vi "PiezoDAQStart.vi"(3 "Waveform":waveform(dbl)={"t0"=timestamp(0 s since 1904-01-01), "dt"=0.0, "Y"=[]}, 10 "error in (no error)":errorcluster) -> (6 "error out":errorcluster)   [LabVIEW 2009]
uses:
  PiezoGlobal.vi
  <vilib>/DAQmx/configure/trigger.llb/DAQmx Start Trigger (Digital Edge).vi
  <vilib>/DAQmx/create/channels.llb/DAQmx Create Channel (CO-Pulse Generation-Time).vi
  <vilib>/DAQmx/configure/timing.llb/DAQmx Timing (Implicit).vi
  <vilib>/DAQmx/write.llb/DAQmx Write (Analog Wfm 1Chan NSamp).vi
  <vilib>/DAQmx/configure/timing.llb/DAQmx Timing (Sample Clock).vi
  <vilib>/DAQmx/create/channels.llb/DAQmx Create Channel (AO-Voltage-Basic).vi
  <vilib>/Waveform/WDTOps.llb/WDT Number of Waveform Samples DBL.vi
  Program Files/National Instruments/LabVIEW 2009/resource/objmgr/daqmx.rc
panel:
  out "True Base Time":dbl format="%.6g"
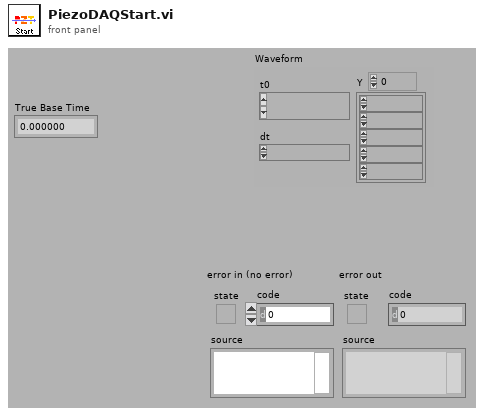
[diagram p1: front panel]
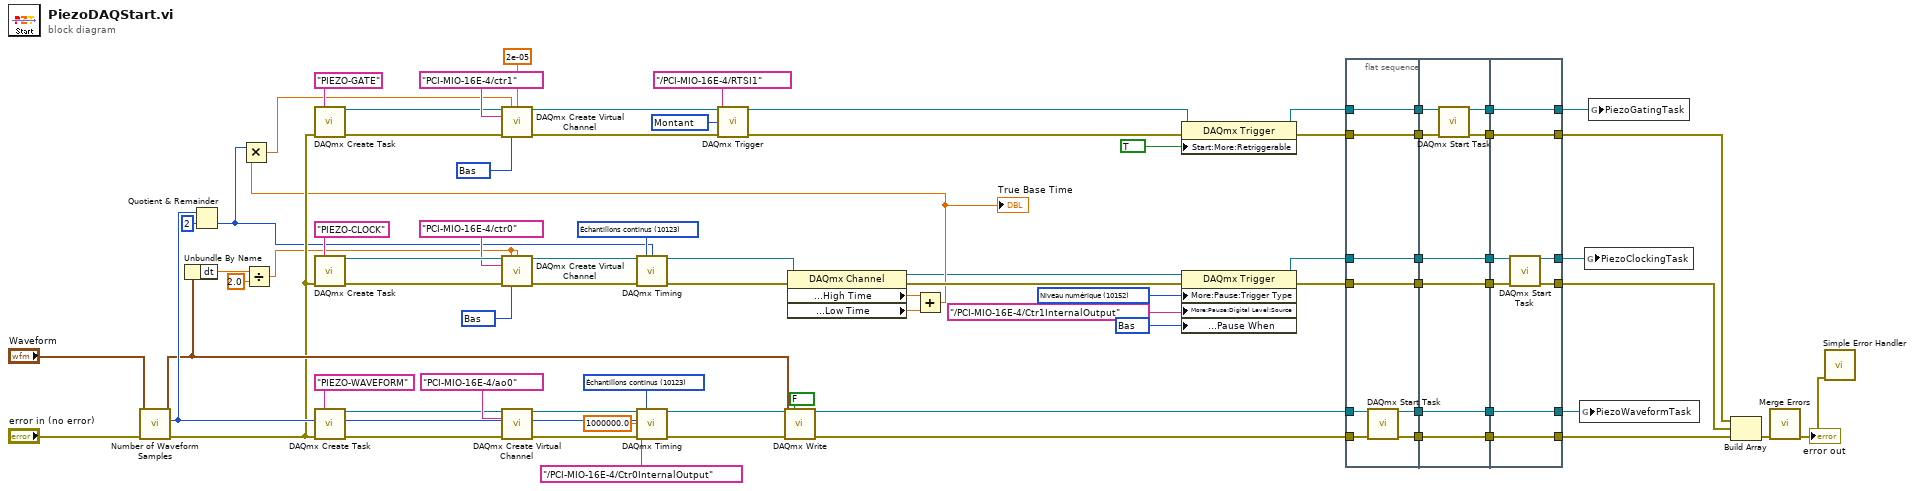
[diagram p0: block diagram]
diagram:
  w32 = 10214 items=["Haut"=10192, "Bas"=10214] ("idle state")
  w33 = 10214 items=["Haut"=10192, "Bas"=10214] ("idle state")
  w38 = 10214 items=["Haut"=10192, "Bas"=10214] ("Pause.NivNum.Lors")
  w39 = 10152 items=["Niveau analogique"=10101, "Fenêtre analogique"=10103, "Niveau numérique"=10152, "Pattern numérique"=10398, "Aucun"=10230] ("Pause.TypeDécl")
  w46 = 10280 items=["Montant"=10280, "Descendant"=10171] ("edge")
  w68 = 10123 items=["Échantillons finis"=10178, "Échantillons continus"=10123, "Point par point avec cadencement matériel"=12522] ("sample mode")
  w77 = 10123 items=["Échantillons finis"=10178, "Échantillons continus"=10123, "Point par point avec cadencement matériel"=12522] ("sample mode")
  n1 = call-poly <vilib>:"Number of Waveform Samples.vi"("error in (no error)"="error in (no error)", "waveform in"="Waveform") -> ("error out"=w36:errorcluster, "number of samples"=w67:i32, "waveform out"=w37:waveform(dbl))  [unwired: 7 in]
  n2 = Unbundle By Name(w37) -> ("dt"=w10:dbl)
  n3 = Quotient & Remainder(x=w67, y=2) -> (floor(x/y)=w19:i32)  [unwired: 1 out]
  n4 = Divide(x=w10, y=2.0) -> (x/y=w8:dbl)
  n5 = call <vilib>:"DAQmx Create Task.vi"("new task name"="PIEZO-GATE", "error in"=w36) -> ("task out"=w50:refnum<k21>, "error out"=w51:errorcluster)  [unwired: 12 in]
  n6 = call <vilib>:"DAQmx Create Task.vi"("new task name"="PIEZO-CLOCK", "error in"=w36) -> ("task out"=w79:refnum<k21>, "error out"=w78:errorcluster)  [unwired: 12 in]
  n7 = call <vilib>:"DAQmx Create Task.vi"("new task name"="PIEZO-WAVEFORM", "error in"=w36) -> ("task out"=w3:refnum<k21>, "error out"=w73:errorcluster)  [unwired: 12 in]
  n8 = call-poly <vilib>:"DAQmx Create Virtual Channel.vi"("task in"=w79, "high time"=w8, "low time"=w8, "counter"=tag "PCI-MIO-16E-4/ctr0", "error in"=w78, "idle state"=w32) -> ("task out"=w57:refnum<k21>, "error out"=w75:errorcluster)  [unwired: 8 in]
  n9 = call-poly <vilib>:"DAQmx Create Virtual Channel.vi"("task in"=w3, "physical channels"=tag "PCI-MIO-16E-4/ao0", "error in"=w73) -> ("task out"=w69:refnum<k21>, "error out"=w70:errorcluster)  [unwired: 11 in]
  n10 = call-poly <vilib>:"DAQmx Timing.vi"("task/channels in"=w57, "sample mode"=w77, "samples per channel"=w19, "error in"=w75) -> ("task out"=w13:refnum<k21>, "error out"=w15:errorcluster)  [unwired: 10 in]
  n11 = call-poly <vilib>:"DAQmx Timing.vi"("task/channels in"=w69, "sample mode"=w68, "samples per channel"=w67, "rate"=1000000.0, "source"=tag "/PCI-MIO-16E-4/Ctr0InternalOutput", "error in"=w70) -> ("task out"=w65:refnum<k21>, "error out"=w66:errorcluster)  [unwired: 8 in]
  n12 = call-poly <vilib>:"DAQmx Write.vi"("task/channels in"=w65, "auto start"=FALSE, "data"=w37, "error in"=w66) -> ("task out"=w1:refnum<k21>, "error out"=w2:errorcluster)  [unwired: 9 in, 1 out]
  n13 = property class="DAQmx Channel"(reference=w13, error in=w15) -> (reference out=w5:refnum<k21>, error out=w14:errorcluster, "Counter Output:Pulse:Time:High Time"=w12:dbl, "Counter Output:Pulse:Time:Low Time"=w11:dbl)
  n14 = Add(x=w12, y=w11) -> (x+y=w7:dbl)
  "True Base Time" <- w7
  n15 = Multiply(x=w19, y=w7) -> (x*y=w18:dbl)
  n16 = call-poly <vilib>:"DAQmx Create Virtual Channel.vi"("task in"=w50, "high time"=w18, "low time"=2e-05, "counter"=tag "PCI-MIO-16E-4/ctr1", "error in"=w51, "idle state"=w33) -> ("task out"=w45:refnum<k21>, "error out"=w47:errorcluster)  [unwired: 8 in]
  n17 = call-poly <vilib>:"DAQmx Trigger.vi"("task/channels in"=w45, "source"=tag "/PCI-MIO-16E-4/RTSI1", "edge"=w46, "error in"=w47) -> ("task out"=w4:refnum<k21>, "error out"=w43:errorcluster)  [unwired: 10 in]
  n18 = property class="DAQmx Trigger"(reference=w4, error in=w43, "Start:More:Retriggerable"=TRUE ("Démarr.Redéclenchable")) -> (reference out=w41:refnum<k21>, error out=w42:errorcluster)
  n19 = property class="DAQmx Trigger"(reference=w5, error in=w14, "More:Pause:Trigger Type"=w39, "More:Pause:Digital Level:Source"=tag "/PCI-MIO-16E-4/Ctr1InternalOutput" ("Pause.NivNum.Src"), "More:Pause:Digital Level:Pause When"=w38) -> (reference out=w54:refnum<k21>, error out=w56:errorcluster)
  n20 = flat-sequence {
    tunnel: w56 -> [w85]
    tunnel: w54 -> [w84]
    tunnel: w2 -> [w88]
    tunnel: [w85] -> w31
    tunnel: [w87] -> w29
    tunnel: w1 -> [w86]
    tunnel: [w84] -> w27
    tunnel: [w83] -> w25
    tunnel: [w82] -> w23
    tunnel: w42 -> [w82]
    tunnel: [w81] -> w21
    tunnel: w41 -> [w81]
    tunnel: w31 -> [w96]
    tunnel: [w96] -> w30
    tunnel: w29 -> [w95]
    tunnel: [w95] -> w28
    tunnel: w27 -> [w94]
    tunnel: [w94] -> w26
    tunnel: w25 -> [w93]
    tunnel: [w93] -> w24
    tunnel: w23 -> [w91]
    tunnel: [w90] -> w22
    tunnel: w21 -> [w92]
    tunnel: [w89] -> w20
    tunnel: [w97] -> w16
    tunnel: [w98] -> w40
    tunnel: [w99] -> w63
    tunnel: [w101] -> w62
    tunnel: [w104] -> w60
    tunnel: [w102] -> w58
    tunnel: w30 -> [w103]
    tunnel: w28 -> [w104]
    tunnel: w26 -> [w100]
    tunnel: w24 -> [w101]
    tunnel: w22 -> [w98]
    tunnel: w20 -> [w97]
    frame #0 {
      n21 = call <vilib>:"DAQmx Start Task.vi"("task/channels in"=w86, "error in"=w88) -> ("task out"=w83:refnum<k21>, "error out"=w87:errorcluster)  [unwired: 12 in]
    }
    frame #1 {
      n22 = call <vilib>:"DAQmx Start Task.vi"("task/channels in"=w92, "error in"=w91) -> ("task out"=w89:refnum<k21>, "error out"=w90:errorcluster)  [unwired: 12 in]
    }
    frame #2 {
      n23 = call <vilib>:"DAQmx Start Task.vi"("task/channels in"=w100, "error in"=w103) -> ("task out"=w99:refnum<k21>, "error out"=w102:errorcluster)  [unwired: 12 in]
    }
  }
  n24 = global write "PiezoGlobal.vi" "PiezoWaveformTask"(w62) -> ()
  n25 = global write "PiezoGlobal.vi" "PiezoClockingTask"(w63) -> ()
  n26 = global write "PiezoGlobal.vi" "PiezoGatingTask"(w16) -> ()
  n27 = Build Array(w40, w58, w60) -> (w59:errorcluster[])
  n28 = call <vilib>:"Merge Errors.vi"("error array in"=w59) -> ("error out"=w61:errorcluster)  [unwired: 6 in]
  "error out" <- w61
  n29 = call <vilib>:"Simple Error Handler.vi"("error in (no error)"=w61) -> ()  [unwired: 4 in, 5 out]
